vi "Initialise.vi"(8 "error in (no error)":errorcluster, 10 "Message in":refnum<class "InitialiseMessage.lvclass">, 11 "AOTF in":refnum<class "Invivo_AOTF.lvclass">) -> (0 "error out":errorcluster, 3 "AOTF out":refnum<class "Invivo_AOTF.lvclass">)   [LabVIEW 2012, in "Invivo_AOTF.lvclass"]
doc: "This method is called when an initialise message is received. It mainly initialises the RabbitMQ connectivity. \n\nOverride this method when your component needs special initialisation (e.g. of software or hardware resources). In that case, don't forget to call the parent for proper implementation. If your component owns subcomponents, they count as resources, so you have to initialise them by calling their own initialise functions"
uses:
  Invivo_AOTF.lvclass
  <vilib>/Distrio/Murmex/InitialiseMessage/InitialiseMessage.lvclass
  <vilib>/Distrio/Murmex/Murmex/Murmex.lvclass
  Invivo_AOTF.lvclass/Invivo_AOTF.ctl
  <vilib>/Instr/_visa.llb/VISA Configure Serial Port (Instr).vi
panel:
  # "This method is called when the INTIALISE\ntrigger is sent. \n\nOverride this method when your component needs to\nrespond to this trigger. \n\nCall parent for proper implementation"
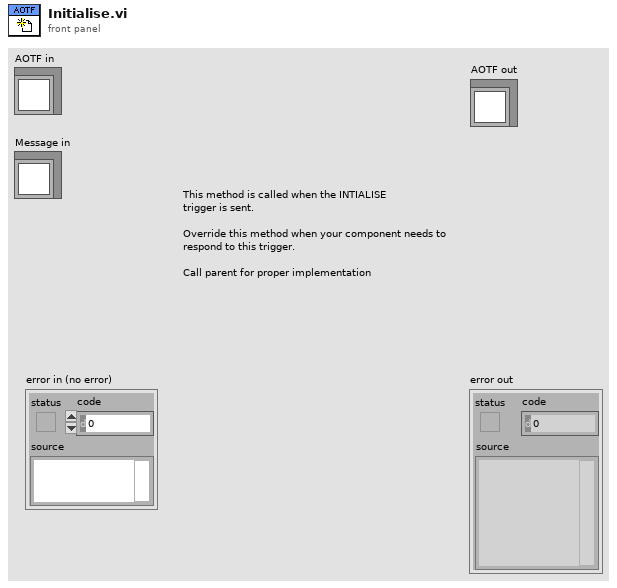
[diagram p1: front panel]
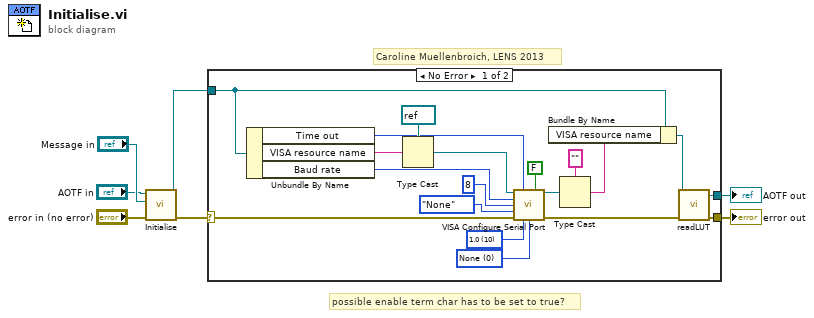
[diagram p0: block diagram]
diagram:
  # "possible enable term char has to be set to true?"
  # "Caroline Muellenbroich, LENS 2013"
  n1 = call-parent "Initialise.vi"("error in (no error)"="error in (no error)", "Message in"="Message in", "Murmex in"="AOTF in") -> ("error out"=w4:errorcluster, "Murmex out"=w3:refnum<class "Invivo_AOTF.lvclass">)  [unwired: 7 in]
  n2 = case shown="No Error" w4 {
    selector: w4 -> [w26 w28]
    tunnel: w3 -> [w9 w27]
    tunnel: [w16 w28] -> w2
    tunnel: [w14 w27] -> w1
    frame No Error {
      w10 = u16 0 items=["None", "XON/XOFF", "RTS/CTS", "XON/XOFF & RTS/CTS", "DTR/DSR", "XON/XOFF & DTR/DSR"] ("flow control (0:none)")
      w13 = u16 10 items=["1.0"=10, "1.5"=15, "2.0"=20] ("stop bits (10: 1 bit)")
      n3 = Unbundle By Name(w9) -> ("Time out"=w18:u32, "VISA resource name"=w23:string, "Baud rate"=w19:u32)
      n4 = Type Cast(type=refnum<visa-resource-name> refnum ("VISA resource name"), x=w23) -> (*(type *) &x=w24:refnum<visa-resource-name>)
      n5 = call-poly "VISA Configure Serial Port"("VISA resource name"=w24, "timeout (10sec)"=w18, "Enable Termination\nChar (T)"=FALSE, "baud rate (9600)"=w19, "data bits (8)"=u16 8, "parity (0:none)"=enum16{"None", "Odd", "Even", "Mark", "Space"}."None", "error in (no error)"=w26, "stop bits (10: 1 bit)"=w13, "flow control (0:none)"=w10) -> ("VISA resource name out"=w22:refnum<visa-resource-name>, "error out"=w17:errorcluster)  [unwired: 5 in]
      n6 = Type Cast(type="" ("Configuration_cluster.VISA resource name"), x=w22) -> (*(type *) &x=w21:string)
      n7 = Bundle By Name(cluster=w9, "VISA resource name"=w21) -> (w15:refnum<class "Invivo_AOTF.lvclass">)
      n8 = call-dynamic "readLUT.vi"("error in (no error)"=w17, "AOTF in"=w15) -> ("error out"=w16:errorcluster, "AOTF out"=w14:refnum<class "Invivo_AOTF.lvclass">)  [unwired: 8 in]
    }
    frame Error {
    }
  }
  "error out" <- w2
  "AOTF out" <- w1
